vi "Shooter Hood.vi"(8 "Hood Position":dbl, 9 "Hood Man. Request?":bool, 10 "Hood Manual Value":dbl, 11 "Shooter States":T2) -> (2 "Shooter Hood Output":dbl, 3 "Hood States To Dashboard":T1)   [LabVIEW 2015]
uses:
  Typedefs/Shooter States.ctl
  Typedefs/Hood States.ctl
panel:
  in  "Shooter Hood Gains":cluster{"kP":dbl, "kI":dbl, "kD":dbl}
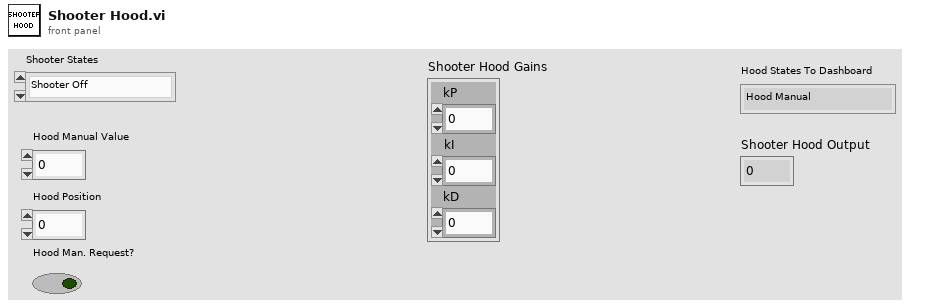
[diagram p1: front panel]
types:
  T1 = typedef "Hood States.ctl" = enum16{"Hood Manual ", "Hood Close Shot", "Hood Far Shot", "Hood Spy Shot", "Hood Intermediate"}
  T2 = typedef "Shooter States.ctl" = enum16{"Shooter Off", "Shooter Far", "Shooter Close", "Shooter Intermediate", "Shooter Spy"}
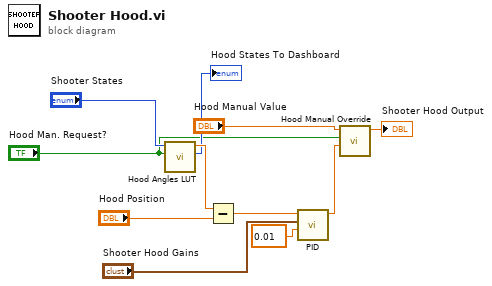
[diagram p0: block diagram]
diagram:
  n1 = call "Hood Angles LUT.vi"("Hood Man Request?"="Hood Man. Request?", "Shooter States"="Shooter States") -> ("Hood States To Dashboard"=→"Hood States To Dashboard":T1, "Hood Angle Setpoint"=w10:dbl)  [unwired: 8 in]
  n2 = Subtract(x=w10, y="Hood Position") -> (x-y=w8:dbl)
  n3 = call "PID.vi"("Loop Period"=0.01, "Gains"="Shooter Hood Gains", "Error"=w8) -> ("Output"=w4:dbl)  [unwired: 6 in, 2 out]
  n4 = call "Hood Manual Override.vi"("Output"=w4, "Hood Man. Request"="Hood Man. Request?", "Hood Manual Value"="Hood Manual Value") -> ("Hood Output"=→"Shooter Hood Output":dbl)  [unwired: 8 in]
